vi "oax_GS Order Power Spectrum (Digital Tacho).vi"(0 "scaled signals [EU]":waveform(dbl)[](array[waveform]), 1 "window type":u32, 2 "block size":i32, 3 "dB On":bool, 5 "digital tacho info":T3={"tacho counts"=[], "counter timebase [Hz]"=1000.0, "counter task type"=enum."event counting", "counter digit (32)"=32}, 7 "Start":dbl, 9 "Duration":dbl, 11 "error in (no error)":errorcluster, 12 "max order to analyze":dbl, 13 "pulse/rev":i32, 14 "averaging parameters":T2) -> (4 "Order Power Spectrum":T1(array[cluster]), 15 "error out":errorcluster)   [LabVIEW 2017]
uses:
  <vilib>/addons/Sound and Vibration/Order Analysis/Tach Process/SubVIs/digital tach info.ctl
  <vilib>/addons/Sound and Vibration/Order Analysis/Resample Order Tracking/OAT Order Power Spectrum (N Channels).vi
  <vilib>/addons/Sound and Vibration/Order Analysis/Resample Order Tracking/OAT Convert to Even Angle Signal (N Channels).vi
  <vilib>/addons/Sound and Vibration/Order Analysis/Tach Process/OAT Digital Tacho Process (1 Tacho).vi
  <vilib>/Waveform/WDTOps.llb/WDT Get Waveform Subset DBL (LV80).vi
  <vilib>/addons/Sound and Vibration/Order Analysis/Resample Order Tracking/SoundVib_OrderTracking.lvlib
  <vilib>/addons/Sound and Vibration/Order Analysis/Tach Process/SoundVib_TachProcess.lvlib
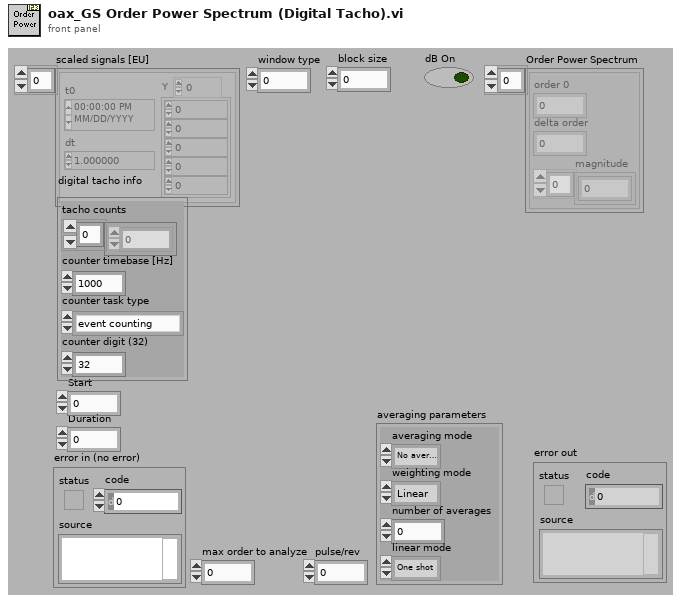
[diagram p1: front panel]
types:
  T1 = cluster{"order 0":dbl, "delta order":dbl, "magnitude":dbl[]}[]
  T2 = cluster{"averaging mode":enum16{"No averaging", "Vector averaging", "RMS averaging", "Peak hold"}, "weighting mode":enum16{"Linear", "Exponential"}, "number of averages":u32, "linear mode":enum16{"One shot", "Auto restart"}}
  T3 = typedef "SoundVib_TachProcess.lvlib/digital tach info.ctl" = cluster{"tacho counts":i64[], "counter timebase [Hz]":dbl, "counter task type":enum16{"period measurement", "event counting"}, "counter digit (32)":i32}
  T4 = typedef "SoundVib_TachProcess.lvlib/speed profile.ctl" = cluster{"time [s]":dbl[], "speed [RPM]":dbl[]}
  T5 = typedef "svc_Resampled Channel Info.ctl" = cluster{"channel name":string, "description":string, " channel info":T6}
  T6 = typedef "svc_Channel Info.ctl" = cluster{"sensor sensitivity":dbl, "engineering units":T7, "dB reference":dbl, "custom label":string, "weighting filter":T8, "pregain":dbl}
  T7 = typedef "svc_Engineering Units Text Ring.ctl" = u16
  T8 = typedef "svc_Weighting Filter Text Ring.ctl" = u16
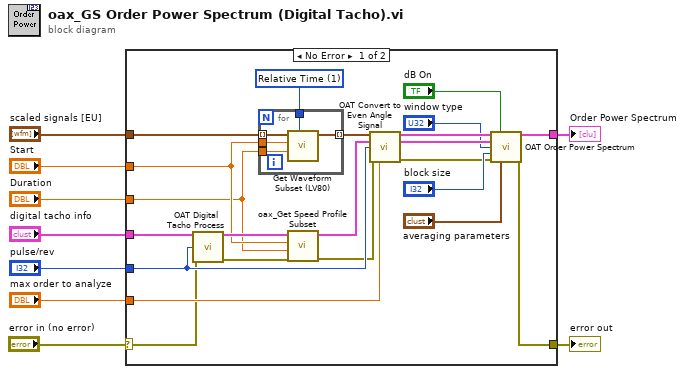
[diagram p0: block diagram]
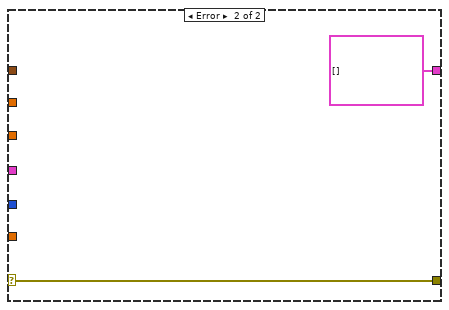
[diagram p2: hidden frame]
diagram:
  n1 = case shown="No Error" "error in (no error)" {
    selector: "error in (no error)" -> [w11 w38]
    tunnel: "scaled signals [EU]" -> [w31 _]
    tunnel: "max order to analyze" -> [w30 _]
    tunnel: [w21 T1 [] ("order power spectrums")] -> w7
    tunnel: "digital tacho info" -> [w20 _]
    tunnel: "pulse/rev" -> [w19 _]
    tunnel: "Start" -> [w13 _]
    tunnel: "Duration" -> [w12 _]
    tunnel: [w10 w38] -> w1
    frame No Error {
      w29 = u16 1 items=["Index", "Relative Time"] ("Mode")
      n2 = call-poly <vilib>:"OAT Digital Tacho Process.vi"("digital tacho info"=w20, "pulse/revolution (1)"=w19, "error in (no error)"=w11) -> ("speed profile"=w18:T4, "error out"=w16:errorcluster)  [unwired: 9 in, 2 out]
      n3 = for {
        tunnel: w13 -> [w36]
        tunnel: w12 -> [w35]
        tunnel: w29 -> [w34]
        tunnel: [w33] -> w26 mode=indexing
        tunnel: w31 -> [w32] mode=indexing
        n4 = call-poly <vilib>:"Get Waveform Subset (LV80).vi"("start/duration format"=w34, "duration"=w35, "start samples/time"=w36, "waveform in"=w32) -> ("waveform out"=w33:waveform(dbl))  [unwired: 2 in, 3 out]
      }
      n5 = call <vilib>:"oax_Get Speed Profile Subset.vi"("error in (no error)"=w16, "Duration"=w12, "Start"=w13, "speed profile"=w18) -> ("error out"=w15:errorcluster, "speed profile out"=w17:T4)  [unwired: 6 in]
      n6 = call-poly <vilib>:"OAT Convert to Even Angle Signal.vi"("scaled signals [EU]"=w26, "speed profile"=w17, "pulse/revolution (1)"=w19, "error in (no error)"=w15, "max order (auto)"=w30) -> ("even-angle signals"=w27:cluster{"r0":dbl, "dr":dbl, "Y":dbl[]}[], "even-angle channel info"=w28:T5[], "error out"=w14:errorcluster)  [unwired: 6 in, 2 out]
      n7 = call-poly <vilib>:"OAT Order Power Spectrum.vi"("even-angle signals"=w27, "dB on? (T)"="dB On", "even-angle channel info"=w28, "window"="window type", "block size"="block size", "error in (no error)"=w14, "averaging parameters"="averaging parameters") -> ("order power spectra"=w21:T1, "error out"=w10:errorcluster)  [unwired: 2 in, 5 out]
    }
    frame Error {
    }
  }
  "Order Power Spectrum" <- w7
  "error out" <- w1
